vi "Confirm Clear Calibration.vi"() -> (3 "clear fs cal?":bool)   [LabVIEW 2020]
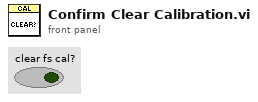
[diagram p1: front panel]
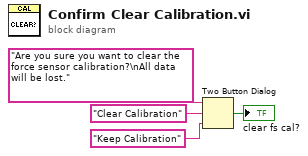
[diagram p0: block diagram]
diagram:
  n1 = Two Button Dialog(message="Are you sure you want to clear the force sensor calibration?\nAll data will be lost.", 1:"Keep Calibration" ("F button name (\"Cancel\")"), 2:"Clear Calibration" ("T button name (\"OK\")")) -> (T button?=→"clear fs cal?":bool)
